vi "Write Element of Delta.vi"(8 "error in (no error)":errorcluster, 9 "Numeric":dbl, 10 "indices":i32[](array[numeric]), 11 "Guidance in":refnum<class "Guidance.lvclass">) -> (0 "error out":errorcluster, 3 "Guidance out":refnum<class "Guidance.lvclass">)   [LabVIEW 2014, in "Guidance Library.lvlib" / "Guidance.lvclass"]
uses:
  Guidance.lvclass
  Guidance.lvclass/Guidance.ctl
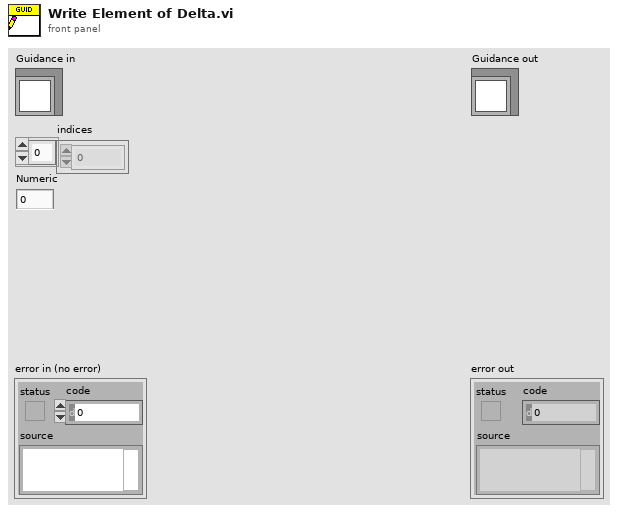
[diagram p1: front panel]
types:
  T1 = typedef "NI_Matrix.lvlib/RealMatrix.ctl" = dbl[][]
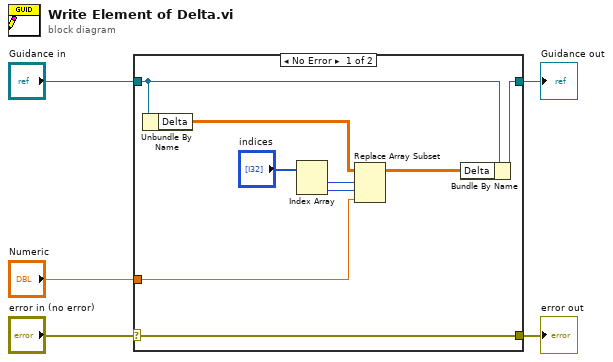
[diagram p0: block diagram]
diagram:
  n1 = case shown="No Error" "error in (no error)" {
    selector: "error in (no error)" -> [w14 w15]
    tunnel: [w14 w15] -> w4
    tunnel: [w13 w16] -> w2
    tunnel: "Guidance in" -> [w6 w16]
    tunnel: "Numeric" -> [w7 _]
    frame No Error {
      n2 = Unbundle By Name(w6) -> ("Delta"=w8:T1)
      n3 = Index Array(array="indices") -> (element #1=w10:i32, element #2=w9:i32)  [unwired: 2 in]
      n4 = Replace Array Subset(array=w8, new element=w7, index (row)=w10, index (col)=w9) -> (w12:T1)
      n5 = Bundle By Name(cluster=w6, "Delta"=w12) -> (w13:refnum<class "Guidance.lvclass">)
    }
    frame Error {
    }
  }
  "error out" <- w4
  "Guidance out" <- w2
